vi "Create Notifiers.vi"(8 "error constant":errorcluster) -> (0 "error out":errorcluster, 2 "output cluster":T1)   [LabVIEW 2017]
uses:
  Notifiers.ctl
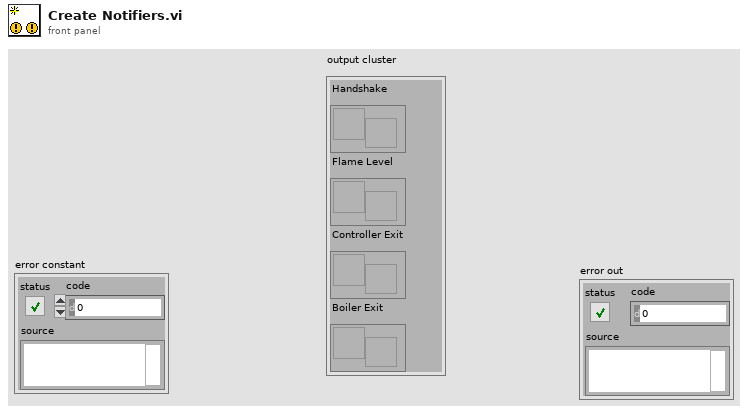
[diagram p1: front panel]
types:
  T1 = typedef "Notifiers.ctl" = cluster{"Handshake":refnum<notifier>, "Flame Level":refnum<notifier>, "Controller Exit":refnum<notifier>, "Boiler Exit":refnum<notifier>}
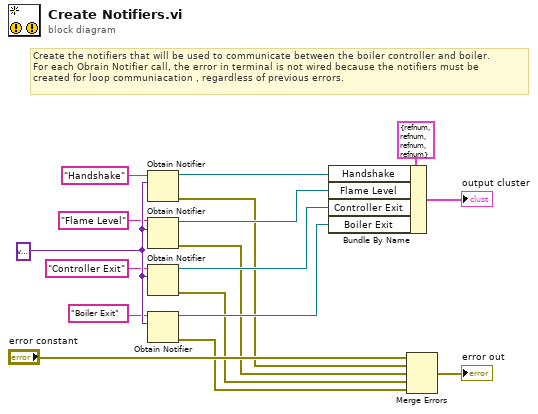
[diagram p0: block diagram]
diagram:
  w17 = variant
  # "Create the notifiers that will be used to communicate between the boiler controller and boiler.\nFor each Obrain Notifier call, the error in terminal is not wired because the notifiers must be \ncreated for loop communiacation , regardless of previous errors."
  n1 = Obtain Notifier(name (unnamed)="Handshake", notification data type=w17) -> (notifier out=w11:refnum<notifier>, error out=w6:errorcluster)  [unwired: 2 in, 1 out]
  n2 = Obtain Notifier(name (unnamed)="Flame Level", notification data type=w17) -> (notifier out=w10:refnum<notifier>, error out=w5:errorcluster)  [unwired: 2 in, 1 out]
  n3 = Obtain Notifier(name (unnamed)="Controller Exit", notification data type=w17) -> (notifier out=w9:refnum<notifier>, error out=w4:errorcluster)  [unwired: 2 in, 1 out]
  n4 = Obtain Notifier(name (unnamed)="Boiler Exit", notification data type=w17) -> (notifier out=w8:refnum<notifier>, error out=w3:errorcluster)  [unwired: 2 in, 1 out]
  n5 = Bundle By Name(cluster=T1 {"Handshake"=refnum, "Flame Level"=refnum, "Controller Exit"=refnum, "Boiler Exit"=refnum}, "Handshake"=w11, "Flame Level"=w10, "Controller Exit"=w9, "Boiler Exit"=w8) -> (→"output cluster":T1)
  n6 = Merge Errors("error constant", w6, w5, w4, w3) -> (→"error out":errorcluster)
